vi "MATLAB Code.vi"(0 "Path_IR":path, 1 "PD_Process":path, 2 "WTW_Process":path, 5 "Path_WTW":path, 9 "D":dbl, 11 "error in (no error)":errorcluster caption="错误输入（无错误）", 12 "K_Process":path, 13 "A_Process":path) -> (4 "a":dbl, 6 "b":dbl, 10 "PD":dbl, 14 "WTW":dbl, 15 "error out":errorcluster caption="错误输出")   [LabVIEW 2015, in "Digital Image Processing.lvlib"]
doc: "该模板用于创建子VI。"
uses:
  Digital Image Processing.lvlib
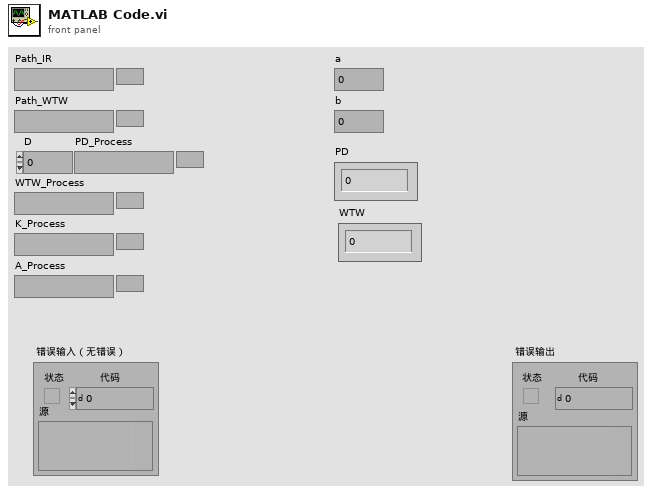
[diagram p1: front panel]
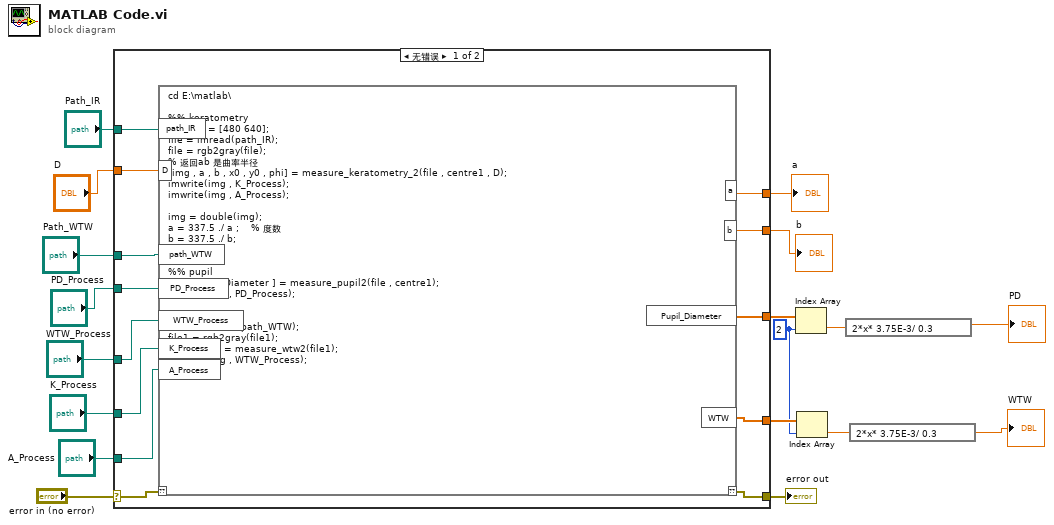
[diagram p0: block diagram]
diagram:
  w9 = 2 ("索引")
  n1 = case shown="无错误" "error in (no error)" {
    selector: "error in (no error)" -> [w31 w32]
    tunnel: [w30 w32] -> w17
    tunnel: "Path_IR" -> [w29 _]
    tunnel: "Path_WTW" -> [w28 _]
    tunnel: "D" -> [w27 _]
    tunnel: [w26 _] -> w13
    tunnel: [w25 _] -> w12
    tunnel: [w24 _] -> w11
    tunnel: [w23 _] -> w10
    tunnel: "PD_Process" -> [w22 _]
    tunnel: "WTW_Process" -> [w21 _]
    tunnel: "K_Process" -> [w20 _]
    tunnel: "A_Process" -> [w19 _]
    frame No Error {
      n2 = script code="cd E:\\matlab\\\n\n%% keratometry\ncentre1 = [480 640];\nfile = imread(path_IR);\nfile = rgb2gray(file);\n% 返回ab 是曲率半径\n[img , a , b , x0 , y0 , phi] = measure_keratometry_2(file , centre1 , D);\nimwrite(img , K_Process);\nimwrite(img , A_Process);\n\nimg = double(img);\na = 337.5 ./ a ;    % 度数\nb = 337.5 ./ b;\n% DD = a-b;\n\n%% pupil \n[ img Pupil_Diameter ] = measure_pupil2(file , centre1);\nimwrite(img , PD_Process);\n\n%% WTW\nfile1 = imread(path_WTW);\nfile1 = rgb2gray(file1);\n[img WTW] = measure_wtw2(file1);\nimwrite(img , WTW_Process);"("??"=w31, "path_IR"=w29, "D"=w27, "path_WTW"=w28, "PD_Process"=w22, "WTW_Process"=w21, "K_Process"=w20, "A_Process"=w19) -> ("??"=w30:errorcluster, "a"=w26:dbl, "b"=w25:dbl, "Pupil_Diameter"=w24:dbl[], "WTW"=w23:dbl[])
    }
    frame Error {
    }
  }
  "error out" <- w17
  "a" <- w13
  "b" <- w12
  n3 = Index Array(array=w11, index=w9) -> (element=w8:dbl)
  n4 = Index Array(array=w10, index=w9) -> (element=w7:dbl)
  n5 = expression code="2*x* 3.75E-3/ 0.3"(w8) -> (→"PD":dbl)
  n6 = expression code="2*x* 3.75E-3/ 0.3"(w7) -> (→"WTW":dbl)
